vi "Find Operations.vi"(8 "error in (no error)":errorcluster caption="entrée d'erreur (pas d'erreur)", 10 "Position":i32, 11 "Operations en entrée":refnum<class "Operations.lvclass"> caption="DNL_LabVIEW Object in") -> (0 "error out":errorcluster caption="sortie d'erreur", 1 "found?":bool, 2 "Parameters":T1, 3 "Operations en sortie":refnum<class "Operations.lvclass"> caption="DNL_LabVIEW Object out")   [LabVIEW 2012, in "Operations.lvclass"]
uses:
  Operations.lvclass
  Operation/Operation Parameters.ctl
  Operation/Operation Type Enum.ctl
  controls/Currencies.ctl
  Operations.lvclass/Operations.ctl
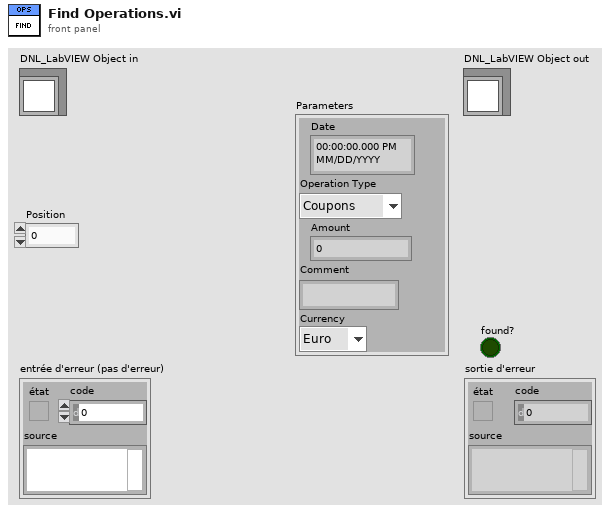
[diagram p1: front panel]
types:
  T1 = typedef "Operation Parameters.ctl" = cluster{"Date":timestamp, "Operation Type":T2, "Amount":dbl, "Comment":string, "Currency":T3}
  T2 = typedef "Operation Type Enum.ctl" = enum16{"Coupons", "Dépot", "Retrait", "Intérêts", "Taxe"}
  T3 = typedef "Currencies.ctl" = enum16{"Euro", "Dollar", "Yen", "RIM", "CHF"}
  T4 = typedef "Dictionary Object RefNum__ogtk.ctl" = refnum<k1>
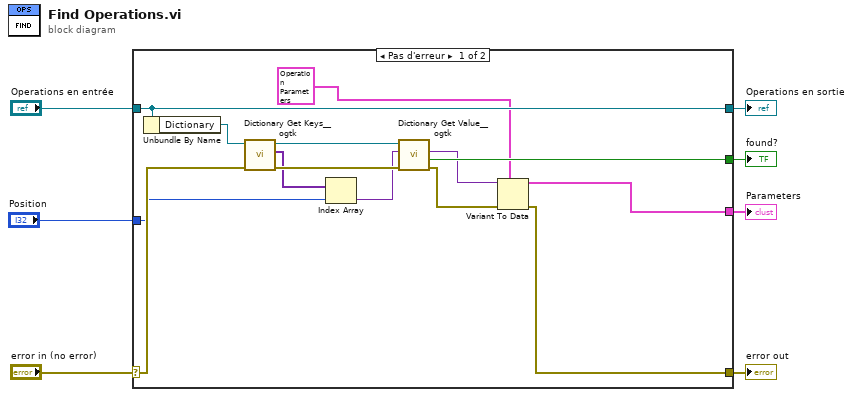
[diagram p0: block diagram]
diagram:
  n1 = case shown="Pas d'erreur" "error in (no error)" {
    selector: "error in (no error)" -> [w14 w23]
    tunnel: [w17 w23] -> w6
    tunnel: [w21 w22] -> w4
    tunnel: "Operations en entrée" -> [w21 w22]
    tunnel: [w20 _] -> w3
    tunnel: "Position" -> [w9 _]
    tunnel: [w15 _] -> w1
    frame No Error {
      n2 = Unbundle By Name(w21) -> ("Dictionary"=w12:T4)
      n3 = call <userlib>:"Dictionary Get Keys__ogtk.vi"("error in (no error)"=w14, "dictionary"=w12) -> ("error out"=w13:errorcluster, "keys"=w10:variant[], "dictionary out"=w11:T4)  [unwired: 7 in]
      n4 = Index Array(array=w10, index=w9) -> (element=w8:variant)
      n5 = call <userlib>:"Dictionary Get Value__ogtk.vi"("error in"=w13, "key"=w8, "dictionary"=w11) -> ("error out"=w18:errorcluster, "found?"=w20:bool, "value"=w19:variant)  [unwired: 5 in, 1 out]
      n6 = Variant To Data(error in=w18, type=T1 {"Date"=timestamp(0 s since 1904-01-01), "Operation Type"=enum."Coupons", "Amount"=0.0, "Comment"="", "Currency"=enum."Euro"} ("Parameters"), Variant=w19) -> (data=w15:T1, error out=w17:errorcluster)
    }
    frame Error {
    }
  }
  "error out" <- w6
  "Operations en sortie" <- w4
  "found?" <- w3
  "Parameters" <- w1
